vi "Autonomous Play Execution.vi"(1 "Input Play":T2) -> (0 "Robot System Functions":T1)   [LabVIEW 2014]
uses:
  Autonomous Play Definition.ctl
  Autonomous Commands/Autonomous Command Names.ctl
  Subsystems VIs/Robot Commands.ctl
  Autonomous Play State.ctl
  Autonomous State global.vi
panel:
  # "Field Centric"
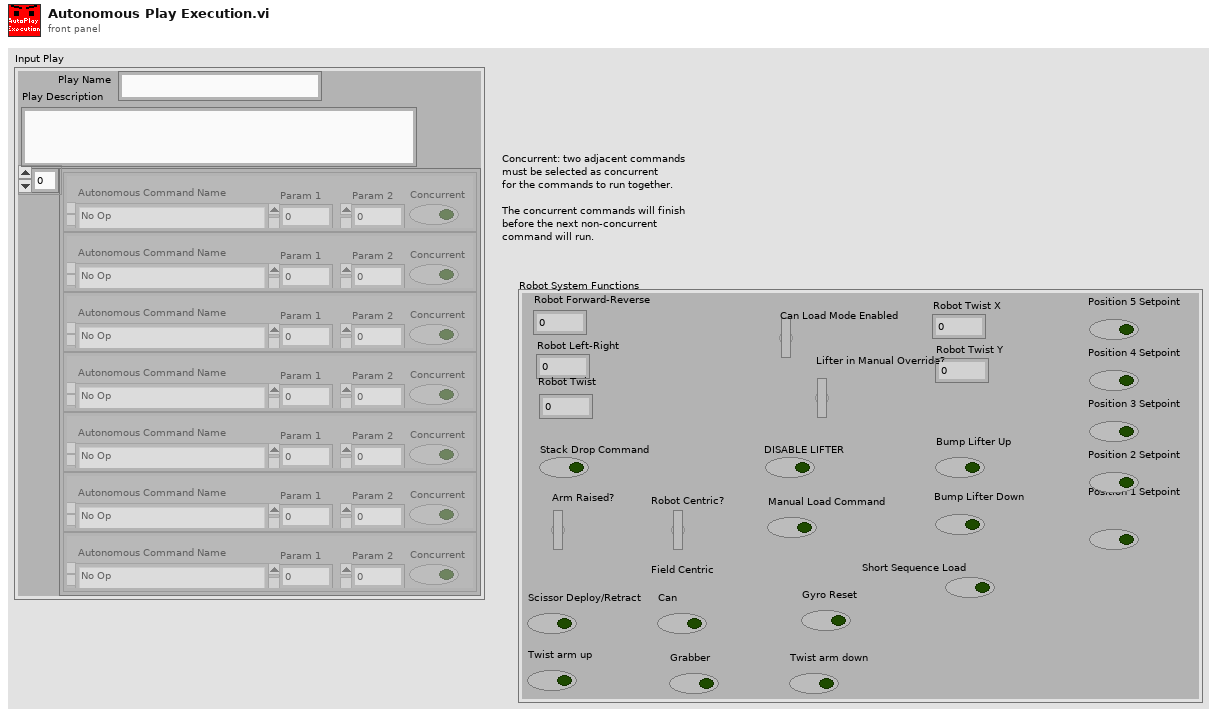
[diagram p1: front panel]
types:
  T1 = typedef "Robot Commands.ctl" = cluster{"Robot Forward-Reverse":dbl, "Robot Left-Right":dbl, "Robot Twist":dbl, "Can Load Mode Enabled":bool, "Lifter in Manual Override?":bool, "Stack Drop Command":bool, "Arm Raised?":bool, "DISABLE LIFTER":bool, "Position 1 Setpoint":bool, "Position 2 Setpoint":bool, "Position 3 Setpoint":bool, "Position 4 Setpoint":bool, "Position 5 Setpoint":bool, "Bump Lifter Down":bool, "Bump Lifter Up":bool, "Manual Load Command":bool, "Robot Centric?":bool, "Scissor Deploy/Retract":bool, "Grabber":bool, "Can":bool, "Twist arm up":bool, "Gyro Reset":bool, "Twist arm down":bool, "Short Sequence Load":bool, "Robot Twist X":dbl, "Robot Twist Y":dbl}
  T2 = typedef "Autonomous Play Definition.ctl" = cluster{"Play Name":string, "Command List":cluster{"Param 1":dbl, "Param 2":dbl, "Autonomous Command Name":T3, "Concurrent":bool}[], "Play Description":string}
  T3 = typedef "Autonomous Command Names.ctl" = enum16{"No Op", "Drive Distance Robot", "Drive Time Robot", "Translate Distance Robot", "Translate Time Robot", "Drive Distance Field", "Drive Time Field", "Translate Distance Field", "Translate Time Field", "Rotate Robot", "Set Initial Gyro Value", "Lifter to Setpoint", "Wait", "Do Not use", "Drive Distance Field (Gyro Hold)", "Translate Distance Field (Gyro Hold)", "Can", "Grabber", "Drive Distance Field (Sensor Stop, Gyro Hold)", "Move Direction Field (Gyro Hold)", "Rotate Robot 90 about Tote", "Reset Gyro", "Find Tote", "Get Tote Into Robot", "Lower Can Grabber"}
  T4 = cluster{"Param 1":dbl, "Param 2":dbl, "Autonomous Command Name":T3, "Concurrent":bool}[]
  T5 = cluster{"Param 1":dbl, "Param 2":dbl, "Autonomous Command Name":T3, "Concurrent":bool}
  T6 = typedef "Autonomous Play State.ctl" = cluster{"Play Name":string, "Autonomous Command Name":T3, "Param 1":dbl, "Param 2":dbl, "Cmd Counter":i32, "Completed":bool}
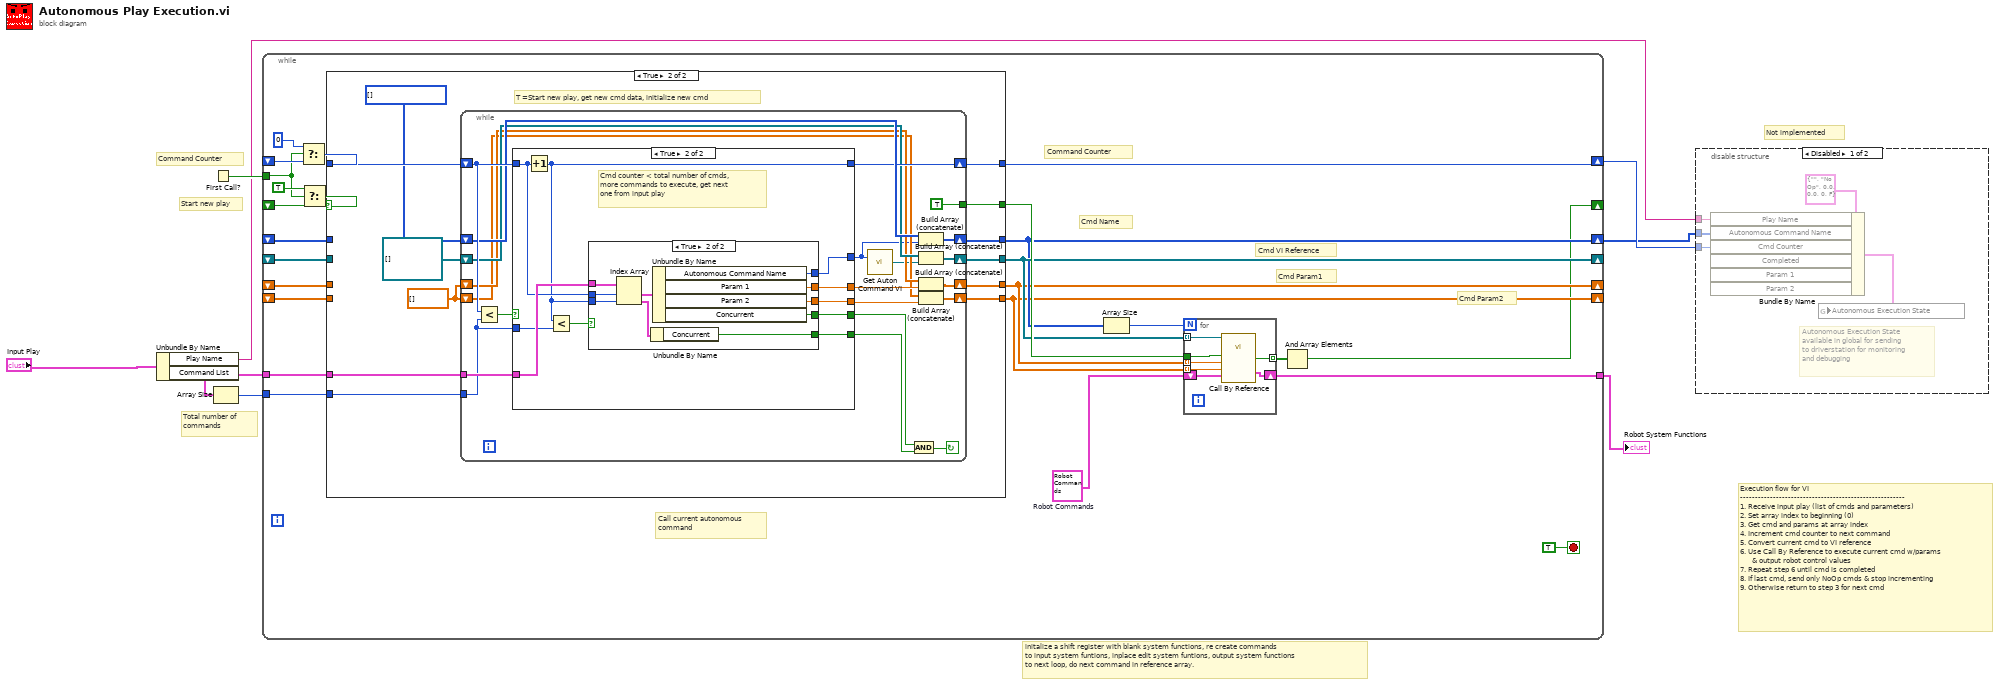
[diagram p0: block diagram]
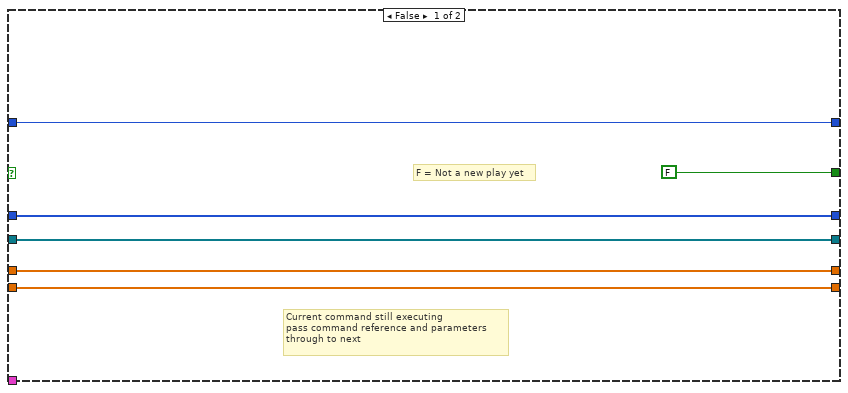
[diagram p3: hidden frame]
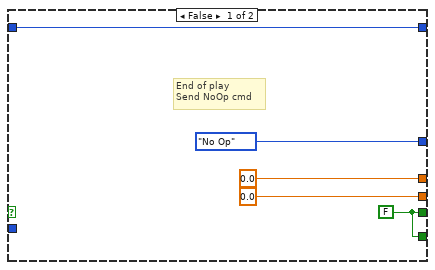
[diagram p4: hidden frame]
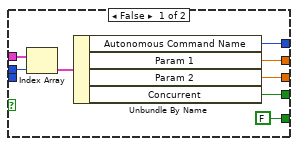
[diagram p5: hidden frame]
diagram:
  # "Not implemented"
  # "initalize a shift register with blank system functions, re create commands\nto input system funtions, inplace edit system funtions, output system functions\nto next loop, do next command in reference array."
  # "Execution flow for VI\n-------------------------------------------------------\n1. Receive input play (list of cmds and parameters)\n2. Set array index to beginning (0)\n3. Get cmd and params at array index\n4. Increment cmd counter to next command\n5. Convert current cmd to VI reference\n6. Use Call By Reference to execute current cmd w/params\n      & output robot control values\n7. Repeat step 6 until cmd is completed\n8. If last cmd, send only NoOp cmds & stop incrementing \n9. Otherwise return to step 3 for next cmd"
  # "Start new play"
  # "Total number of \ncommands"
  # "Command Counter"
  n1 = Unbundle By Name("Input Play") -> ("Play Name"=w1:string, "Command List"=w5:T4)
  n2 = First Call?() -> (First Call?: T/F=w4:bool)
  n3 = Array Size(array=w5) -> (size(s)=w7:i32)
  n4 = while {
    tunnel: w5 -> [w31]
    tunnel: w7 -> [w28]
    shift-right: [w30] -> w6
    shift-left: _ -> [w24]
    shift-right: [w12] -> _
    shift-left: _ -> [w22]
    shift-right: [w15] -> _
    shift-left: _ -> [w18]
    shift-right: [w32] -> _
    shift-left: _ -> [w13]
    shift-right: [w14] -> _
    shift-left: _ -> [w19]
    shift-right: [w17] -> w3
    shift-left: _ -> [w27]
    tunnel: w4 -> [w20]
    tunnel: [w9] -> w2
    stop <- TRUE stop-if-true
    w10 = T1 {"Robot Forward-Reverse"=0.0, "Robot Left-Right"=0.0, "Robot Twist"=0.0, "Can Load Mode Enabled"=FALSE, "Lifter in Manual Override?"=FALSE, "Stack Drop Command"=FALSE, "Arm Raised?"=FALSE, "DISABLE LIFTER"=FALSE, "Position 1 Setpoint"=FALSE, "Position 2 Setpoint"=FALSE, "Position 3 Setpoint"=FALSE, "Position 4 Setpoint"=FALSE, "Position 5 Setpoint"=FALSE, "Bump Lifter Down"=FALSE, "Bump Lifter Up"=FALSE, "Manual Load Command"=FALSE, "Robot Centric?"=FALSE, "Scissor Deploy/Retract"=FALSE, "Grabber"=FALSE, "Can"=FALSE, "Twist arm up"=FALSE, "Gyro Reset"=FALSE, "Twist arm down"=FALSE, "Short Sequence Load"=FALSE, "Robot Twist X"=0.0, "Robot Twist Y"=0.0}  # Robot Commands
    # "Cmd Name"
    # "Cmd Param2"
    # "Cmd Param1"
    # "Cmd VI Reference"
    # "Command Counter"
    # "Call current autonomous\ncommand"
    n5 = Select(t=0, s=w20, f=w24) -> (s? t:f=w25:i32)
    n6 = Select(t=TRUE, s=w20, f=w22) -> (s? t:f=w26:bool)
    n7 = case shown="True" w26 {
      tunnel: w31 -> [_ w58]
      tunnel: w25 -> [w46 w54]
      tunnel: [w44 w57] -> w14
      tunnel: [w43 w56] -> w15
      tunnel: [w46 w52] -> w30
      tunnel: [FALSE w55] -> w33
      tunnel: w28 -> [_ w53]
      tunnel: w27 -> [w42 _]
      tunnel: w19 -> [w44 _]
      tunnel: w18 -> [w43 _]
      tunnel: [w41 w51] -> w32
      tunnel: [w42 w50] -> w17
      tunnel: w13 -> [w41 _]
      frame False {
        # "F = Not a new play yet"
        # "Current command still executing\npass command reference and parameters \nthrough to next"
      }
      frame True {
        w48 = T3[] [] items=["No Op", "Drive Distance Robot", "Drive Time Robot", "Translate Distance Robot", "Translate Time Robot", "Drive Distance Field", "Drive Time Field", "Translate Distance Field", "Translate Time Field", "Rotate Robot", "Set Initial Gyro Value", "Lifter to Setpoint", "Wait", "Do Not use", "Drive Distance Field (Gyro Hold)", "Translate Distance Field (Gyro Hold)", "Can", "Grabber", "Drive Distance Field (Sensor Stop, Gyro Hold)", "Move Direction Field (Gyro Hold)", "Rotate Robot 90 about Tote", "Reset Gyro", "Find Tote", "Get Tote Into Robot", "Lower Can Grabber"]
        w49 = dbl[] []
        # "T =Start new play, get new cmd data, initialize new cmd"
        n8 = while {
          tunnel: w58 -> [w77]
          tunnel: [TRUE] -> w55
          tunnel: w53 -> [w63]
          shift-right: [w74] -> w52
          shift-left: w54 -> [w79]
          shift-right: [w61] -> w51
          shift-left: refnum<vi>[] [] -> [w73]
          shift-right: [w72] -> w56
          shift-left: w49 -> [w70]
          shift-right: [w69] -> w57
          shift-left: w49 -> [w68]
          shift-right: [w66] -> w50
          shift-left: w48 -> [w78]
          stop <- w65 continue-if-true
          n9 = Less?(x=w79, y=w63) -> (x < y?=w75:bool)
          n10 = case shown="True" w75 {
            tunnel: w77 -> [_ w94]
            tunnel: [0.0 ("Param 2") w93] -> w67
            tunnel: [0.0 ("Param 1") w92] -> w71
            tunnel: w79 -> [w82 w91]
            tunnel: [w82 w85] -> w74
            tunnel: [Autonomous_Command_Names."No Op" ("Autonomous Command Name") w90] -> w59
            tunnel: [w80 w89] -> w64
            tunnel: w63 -> [_ w88]
            tunnel: [w80 w86] -> w62
            frame False {
              w80 = FALSE ("Concurrent")
              # "End of play\nSend NoOp cmd"
            }
            frame True {
              # "Cmd counter < total number of cmds,\nmore commands to execute, get next\none from input play"
              n11 = Increment(x=w91) -> (x+1=w85:i32)
              n12 = Less?(x=w85, y=w88) -> (x < y?=w87:bool)
              n13 = case shown="True" w87 {
                tunnel: w94 -> [w95 w112]
                tunnel: [w100 w111] -> w93
                tunnel: [w99 w110] -> w92
                tunnel: w91 -> [w96 w109]
                tunnel: [w98 w108] -> w90
                tunnel: [w101 w107] -> w89
                tunnel: [FALSE ("Concurrent") w105] -> w86
                tunnel: w85 -> [_ w104]
                frame False {
                  n14 = Index Array(array=w95, index=w96) -> (element=w97:T5)
                  n15 = Unbundle By Name(w97) -> ("Autonomous Command Name"=w98:T3, "Param 1"=w99:dbl, "Param 2"=w100:dbl, "Concurrent"=w101:bool)
                }
                frame True {
                  n16 = Index Array(array=w112, index #1=w109, index #2=w104) -> (element #1=w106:T5, element #2=w103:T5)
                  n17 = Unbundle By Name(w103) -> ("Concurrent"=w105:bool)
                  n18 = Unbundle By Name(w106) -> ("Autonomous Command Name"=w108:T3, "Param 1"=w110:dbl, "Param 2"=w111:dbl, "Concurrent"=w107:bool)
                }
              }
            }
          }
          n19 = call "Get Auton Command VI.vi"("Autonomous Command Name"=w59) -> ("VI Refnum"=w60:refnum<vi>)
          n20 = And(x=w64, y=w62) -> (x .and. y?=w65:bool)
          n21 = Build Array (concatenate)(w78, w59) -> (w66:T3[])
          n22 = Build Array (concatenate)(w73, w60) -> (w61:refnum<vi>[])
          n23 = Build Array (concatenate)(w70, w71) -> (w72:dbl[])
          n24 = Build Array (concatenate)(w68, w67) -> (w69:dbl[])
        }
      }
    }
    n25 = Array Size(array=w17) -> (size(s)=w16:i32)
    n26 = for {
      N: w16 -> [_]
      tunnel: w32 -> [w39] mode=indexing
      tunnel: w15 -> [w35] mode=indexing
      tunnel: w14 -> [w36] mode=indexing
      tunnel: w33 -> [w34]
      shift-right: [w37] -> w9
      shift-left: w10 -> [w40]
      tunnel: [w38] -> w11 mode=indexing
      n27 = call-by-ref "?"(reference=w39, "Input Robot System Funtions"=w40, "Cmd Parameter 1"=w36, "Cmd Parameter 2"=w35, "Startup"=w34) -> ("Output Robot System Functions"=w37:T1, "Completed"=w38:bool)  [unwired: 1 in, 2 out]
    }
    n28 = And Array Elements(Boolean array=w11) -> (logical AND=w12:bool)
  }
  "Robot System Functions" <- w2
  n29 = disable-structure shown="Disabled" {
    disable-tunnel: w6 -> [w115 _]
    disable-tunnel: w1 -> [w114 _]
    disable-tunnel: w3 -> [w113 _]
    frame Disabled {
      # "Autonomous Execution State\navailable in global for sending\nto driverstation for monitoring\nand debugging"
      n30 = Bundle By Name(cluster=T6 {"Play Name"="", "Autonomous Command Name"=enum."No Op", "Param 1"=0.0, "Param 2"=0.0, "Cmd Counter"=0, "Completed"=FALSE} ("Autonomous Execution State"), "Play Name"=w114, "Autonomous Command Name"=w113, "Cmd Counter"=w115) -> (w116:T6)  [unwired: 3 in]
      n31 = global write "Autonomous State global.vi" "Autonomous Execution State"(w116) -> ()
    }
    frame Enabled {
    }
  }
